vi "RequestHorizontal.vi"(7 "check postion of these axes":T1[](array[typedef]), 8 "error in (no error)":errorcluster, 9 "Motion Config":bool=TRUE, 11 "MotionComm in":refnum<class "MotionComm.lvclass">) -> (0 "error out":errorcluster, 1 "Horizontal polarization position":dbl, 3 "MotionComm out":refnum<class "MotionComm.lvclass">)   [LabVIEW 2019, in "MotionComm.lvclass"]
uses:
  MotionComm.lvclass
  APARMainSubvis/VXM Public API/mmWaveAxis.ctl
  MotionComm.lvclass/MotionComm.ctl
  Support/MessageQue/MessageQue.lvlib
panel:
  # "^ always using 1 for horizontal definition"
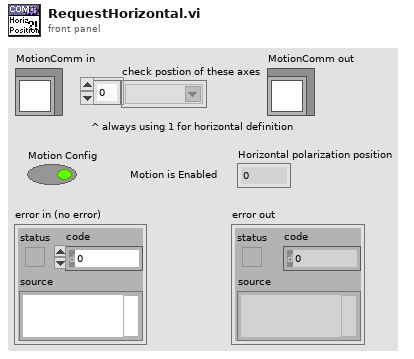
[diagram p1: front panel]
types:
  T1 = typedef "mmWaveAxis.ctl" = string
  T2 = typedef "MessageQue.lvlib/MessageQue.ctl" = refnum<queue>
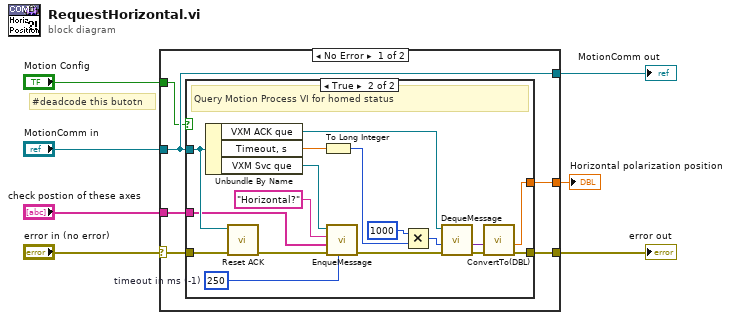
[diagram p0: block diagram]
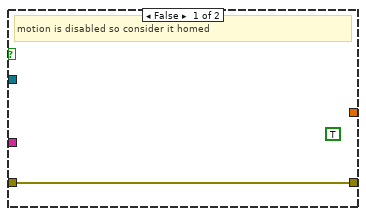
[diagram p2: hidden frame]
diagram:
  # "#deadcode this butotn"
  n1 = case shown="No Error" "error in (no error)" {
    selector: "error in (no error)" -> [w12 w33]
    tunnel: [w11 w33] -> w6
    tunnel: [w13 w32] -> w4
    tunnel: "MotionComm in" -> [w13 w32]
    tunnel: "Motion Config" -> [w10 _]
    tunnel: "check postion of these axes" -> [w9 _]
    tunnel: [w8 _] -> w1
    frame No Error {
      n2 = case shown="True" w10 {
        tunnel: w13 -> [_ w26]
        tunnel: w12 -> [w14 w24]
        tunnel: [w14 w23] -> w11
        tunnel: w9 -> [_ w17]
        tunnel: [_ w15] -> w8
        frame False {
          (unwired) TRUE ("Message Payload boolean")
          # "motion is disabled so consider it homed"
        }
        frame True {
          w16 = 250  # timeout in ms (-1)
          # "Query Motion Process VI for homed status"
          n3 = Unbundle By Name(w26) -> ("VXM ACK que"=w27:T2, "Timeout, s"=w28:dbl, "VXM Svc que"=w21:T2)
          n4 = call "Reset ACK.vi"("error in (no error)"=w24, "MotionComm in"=w26) -> ("error out"=w20:errorcluster)  [unwired: 8 in, 1 out]
          n5 = To Long Integer(number=w28) -> (32bit integer=w30:i32)
          n6 = call "EnqueMessage.vi"("timeout in ms (-1)"=w16, "error in"=w20, "Message Payload"=w17, "Message Command"="Horizontal?", "Message que"=w21) -> ("error out"=w19:errorcluster)  [unwired: 5 in, 1 out]
          n7 = Multiply(x=1000 ("timeout in ms (-1)"), y=w30) -> (x*y=w29:i32)
          n8 = call "DequeMessage.vi"("error in"=w19, "timeout in ms (-1)"=w29, "Message que"=w27) -> ("error out"=w22:errorcluster, "Message Payload"=w25:variant)  [unwired: 3 in, 4 out]
          n9 = call "ConvertTo(DBL).vi"("error in"=w22, "Message Payload"=w25) -> ("error out"=w23:errorcluster, "Message Payload DBL Numeric"=w15:dbl)  [unwired: 8 in]
        }
      }
    }
    frame Error {
    }
  }
  "error out" <- w6
  "MotionComm out" <- w4
  "Horizontal polarization position" <- w1
